vi "Format Current Source String.vi"(9 "Item Count":i32, 11 "Current Path":path) -> (3 "Current Source String":string)   [LabVIEW 2020, in "VI Properties Editor.lvlib"]
doc: "Formats the Current Source string using the provided inputs."
uses:
  VI Properties Editor.lvlib
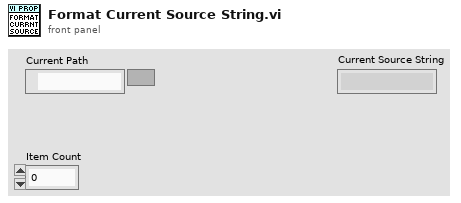
[diagram p1: front panel]
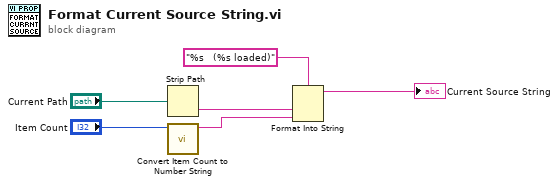
[diagram p0: block diagram]
diagram:
  n1 = Strip Path(path="Current Path") -> (name=w2:string)  [unwired: 1 out]
  n2 = call "Convert Item Count to Number String.vi"("Item Count"="Item Count") -> ("Number of Items String"=w1:string)  [unwired: 10 in]
  n3 = Format Into String(format string="%s   (%s loaded)", w2, w1) -> (resulting string=→"Current Source String":string)  [unwired: 2 in, 1 out]
